vi "RunMainAsync.vi"(3 "ROS_Master.lvclass in":refnum<class "ROS_Master.lvclass">) -> ()   [LabVIEW 2013]
uses:
  <userlib>/ROSforLV/ROS/Code/SubVIs/ROS_Master/ROS_Master.lvclass
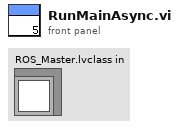
[diagram p1: front panel]
types:
  T1 = enum32{"Bad", "Idle", "Run top level", "Running"}
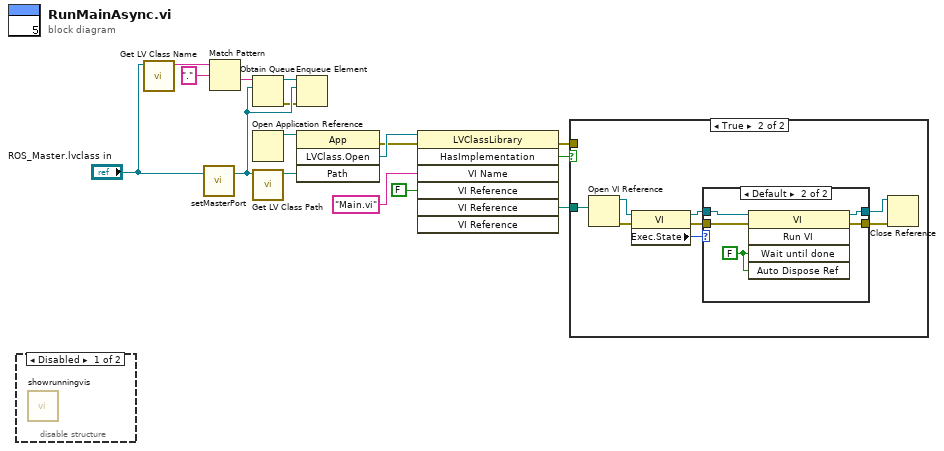
[diagram p0: block diagram]
diagram:
  n1 = disable-structure shown="Disabled" {
    frame Disabled {
      n2 = call <userlib>:"showrunningvis.vi"() -> ()  [unwired: 1 in]
    }
    frame Enabled {
    }
  }
  n3 = call <vilib>:"Get LV Class Name.vi"("object"="ROS_Master.lvclass in") -> ("class name"=w6:string)  [unwired: 9 in, 1 out]
  n4 = call <userlib>:"setMasterPort.vi"("ROS_Master.lvclass in"="ROS_Master.lvclass in") -> ("ROS_Master.lvclass out"=w2:refnum<class "ROS_Master.lvclass">)  [unwired: 2 in]
  n5 = Match Pattern(string=w6, regular expression=".") -> (after substring=w4:string)  [unwired: 1 in, 3 out]
  n6 = Obtain Queue(name (unnamed)=w4, element data type=w2) -> (queue out=w3:refnum<queue>, error out=w1:errorcluster)  [unwired: 3 in, 1 out]
  n7 = Open Application Reference() -> (3:w11:refnum<vi>)  [unwired: 4 in, 1 out]
  n8 = call <vilib>:"Get LV Class Path.vi"("object"=w2) -> ("class path"=w8:path)  [unwired: 9 in, 1 out]
  n9 = Enqueue Element(queue=w3, element=w2, error in (no error)=w1) -> ()  [unwired: 1 in, 3 out]
  n10 = invoke class="App" method="LVClass.Open"(reference=w11, "Path"=w8) -> (error out=w9:errorcluster, "LVClass.Open"=w10:refnum<vi>)  [unwired: 2 in, 2 out]
  n11 = invoke class="LVClassLibrary" method="HasImplementation"(reference=w10, error in=w9, "VI Name"="Main.vi", "VI Reference"=FALSE ("Consider Parent Classes?")) -> (error out=w12:errorcluster, "HasImplementation"=w15:bool, "VI Reference"=w14:path)  [unwired: 3 in, 4 out]
  n12 = case shown="True" w15 {
    tunnel: w14 -> [_ w24]
    tunnel: w12 -> [_ _]
    frame False {
    }
    frame True {
      n13 = Open VI Reference(vi path=w24) -> (vi reference=w17:refnum<vi>, error out=w23:errorcluster)  [unwired: 5 in]
      n14 = property class="VI"(reference=w17, error in=w23) -> (reference out=w21:refnum<vi>, error out=w20:errorcluster, "Exec.State"=w22:T1)
      n15 = case shown="Default" w22 {
        tunnel: w21 -> [w26 w31]
        tunnel: w20 -> [w25 w30]
        tunnel: [w26 w28] -> w19
        tunnel: [w25 w27] -> w18
        frame "Run top level", "Running" {
        }
        frame Default {
          w29 = FALSE ("Wait Until Done")
          n16 = invoke class="VI" method="Run VI"(reference=w31, error in=w30, "Wait until done"=w29, "Auto Dispose Ref"=w29) -> (reference out=w28:refnum<vi>, error out=w27:errorcluster)  [unwired: 1 in, 3 out]
        }
      }
      n17 = Close Reference(reference=w19, error in (no error)=w18) -> ()  [unwired: 1 out]
    }
  }
